vi "Read Inputs from system.vi"(8 "error in":errorcluster, 11 "fixed channel tag bus module in":refnum<class "user control module.lvclass">) -> (0 "error out":errorcluster, 2 "Inputs from system":T1, 3 "fixed channel tag bus module out":refnum<class "user control module.lvclass">)   [LabVIEW 2013, in "user control module.lvclass"]
uses:
  user control module.lvclass
  configuration/input data indices.ctl
  configuration/user control module configuration.lvclass
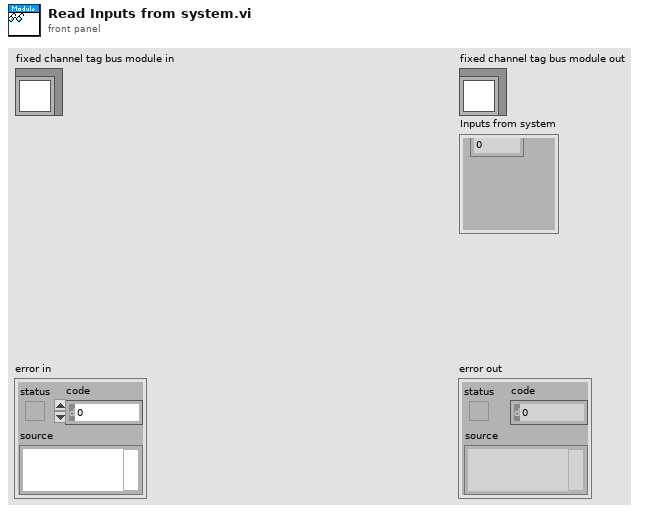
[diagram p1: front panel]
types:
  T1 = typedef "user control module configuration.lvclass/input data indices.ctl" = cluster{"Single.placeholder":i32}
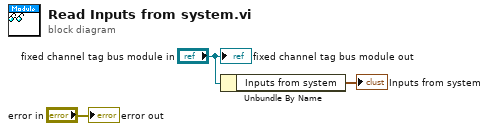
[diagram p0: block diagram]
diagram:
  n1 = Unbundle By Name("fixed channel tag bus module in") -> ("Inputs from system"=→"Inputs from system":T1)
  "error out" <- "error in"
  "fixed channel tag bus module out" <- "fixed channel tag bus module in"
